vi "PPMS.setMagnet.vi"(8 "error in (no error)":errorcluster, 10 "Data":variant, 11 "instrument.PPMS":refnum<class "instrument.PPMS.lvclass">) -> (0 "error out":errorcluster, 3 "instrument.PPMS out":refnum<class "instrument.PPMS.lvclass">)   [LabVIEW 2019, in "instrument.PPMS.lvclass"]
uses:
  instrument.PPMS.lvclass
  <userlib>/LevyLab/Instrument Framework/Instrument Types/Cryostat/Typedefs/setMagnet--cluster.ctl
  <userlib>/LevyLab/Instrument Framework/Instrument Types/Cryostat/Typedefs/Magnet Axis--Enum.ctl
  <userlib>/LevyLab/Instrument Framework/Instrument Types/Cryostat/Typedefs/Magnet Mode--Enum.ctl
  instrument.PPMS.lvclass/instrument.PPMS.ctl
  a0402abb-d6b5-47cd-a717-1b1f96a498df.vi
  <vilib>/JDP Science/JSONtext/JSON text to Variant.vi
  <vilib>/JDP Science/JSONtext/LVClass Serializer/JSONtext LVClass Serializer.lvclass
  <userlib>/LevyLab/Instrument Framework/Instrument Types/Cryostat/Instrument.Cryostat.lvclass
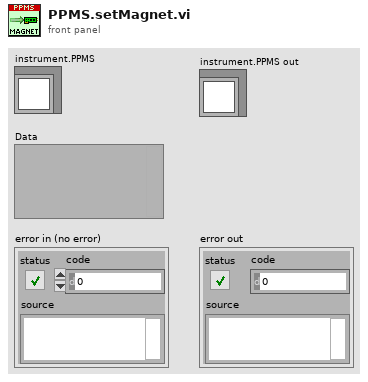
[diagram p1: front panel]
types:
  T1 = typedef "Instrument.Cryostat.lvclass/setMagnet--cluster.ctl" = cluster{"field":dbl, "rate":dbl, "axis":T2, "mode":T3}
  T2 = typedef "Instrument.Cryostat.lvclass/Magnet Axis--Enum.ctl" = enum16{"X", "Y", "Z"}
  T3 = typedef "Instrument.Cryostat.lvclass/Magnet Mode--Enum.ctl" = enum16{"Persistent", "Driven"}
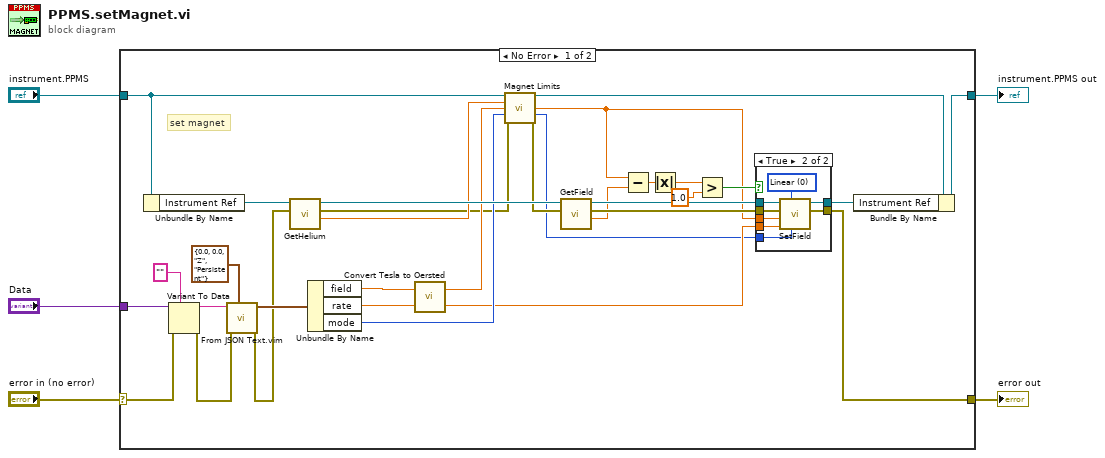
[diagram p0: block diagram]
diagram:
  n1 = case shown="No Error" "error in (no error)" {
    selector: "error in (no error)" -> [w21 w49]
    tunnel: "Data" -> [w22 _]
    tunnel: [w11 w49] -> w4
    tunnel: "instrument.PPMS" -> [w9 w48]
    tunnel: [w12 w48] -> w1
    frame No Error {
      # "set magnet"
      n2 = Unbundle By Name(w9) -> ("Instrument Ref"=w31:refnum<k24>)
      n3 = Variant To Data(error in=w21, type="", Variant=w22) -> (data=w24:string, error out=w20:errorcluster)
      n4 = call "From JSON Text.vim"("Data Type and Default Value"=T1 {"field"=0.0, "rate"=0.0, "axis"=enum."Z", "mode"=enum."Persistent"} ("Set Magnet Field"), "error in (no error)"=w20, "JSON"=w24) -> ("error out"=w19:errorcluster, "Data out"=w23:T1)  [unwired: 7 in]
      n5 = call "GetHelium.vi"("error in (no error)"=w19, "Instrument Refnum in"=w31) -> ("Helium Level (%)"=w27:dbl, "error out"=w8:errorcluster, "Instrument Ref Out"=w30:refnum<k24>)  [unwired: 3 in]
      n6 = Unbundle By Name(w23) -> ("field"=w17:dbl, "rate"=w16:dbl, "mode"=w15:T3)
      n7 = call "Convert Tesla to Oersted.vi"("Field Rate (T/min)"=w16, "Field (T)"=w17) -> ("Field Rate (Oe/s)"=w10:dbl, "Field (Oe)"=w26:dbl)
      n8 = call-dynamic "Magnet Limits.vi"("instrument.PPMS"=w9, "Helium (%)"=w27, "Target Field (Oe)"=w26, "Mode"=w15, "error in (no error)"=w8) -> ("instrument.PPMS out"=w13:refnum<class "instrument.PPMS.lvclass">, "Limited Field (Oe)"=w28:dbl, "Mode out"=w6:T3, "error out"=w7:errorcluster)  [unwired: 7 in]
      n9 = call "GetField.vi"("error in (no error)"=w7, "Instrument Ref In"=w30) -> ("Field"=w29:dbl, "error out"=w37:errorcluster, "Instrument Ref Out"=w36:refnum<k24>)  [unwired: 3 in, 2 out]
      n10 = Subtract(x=w28, y=w29) -> (x-y=w33:dbl)
      n11 = Absolute Value(x=w33) -> (abs(x)=w35:dbl)
      n12 = Greater?(x=w35, y=1.0) -> (0:w32:bool)
      n13 = case shown="True" w32 {
        tunnel: [w39 w46] -> w11
        tunnel: w37 -> [w39 w45]
        tunnel: w36 -> [w38 w44]
        tunnel: w28 -> [_ w43]
        tunnel: w6 -> [_ w42]
        tunnel: w10 -> [_ w41]
        tunnel: [w38 w40] -> w14
        frame False {
        }
        frame True {
          w47 = 0 items=["Linear", "NoOvershoot", "Oscillate"] ("Approach")
          n14 = call "SetField.vi"("Mode"=w42, "Approach"=w47, "Rate"=w41, "Field"=w43, "error in (no error)"=w45, "Instrument Ref In"=w44) -> ("error out"=w46:errorcluster, "Instrument Ref Out"=w40:refnum<k24>)  [unwired: 1 in, 1 out]
        }
      }
      n15 = Bundle By Name(cluster=w13, "Instrument Ref"=w14) -> (w12:refnum<class "instrument.PPMS.lvclass">)
    }
    frame Error {
    }
  }
  "error out" <- w4
  "instrument.PPMS out" <- w1
